vi "C37 Get PMU Configuration.vi"(8 "error in (no error)":errorcluster, 10 "PMU Index":i32, 11 "Pseudo PDC ID":i32) -> (0 "error out":errorcluster, 2 "Station Name":string, 3 "PMU Configuration":T1)   [LabVIEW 2013, in "C37118-DLL.lvlib"]
uses:
  C37118-DLL.lvlib
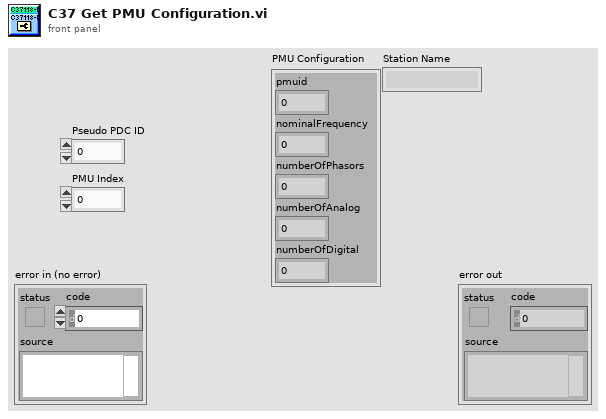
[diagram p1: front panel]
types:
  T1 = cluster{"pmuid":i32, "nominalFrequency":sgl, "numberOfPhasors":i32, "numberOfAnalog":i32, "numberOfDigital":i32}
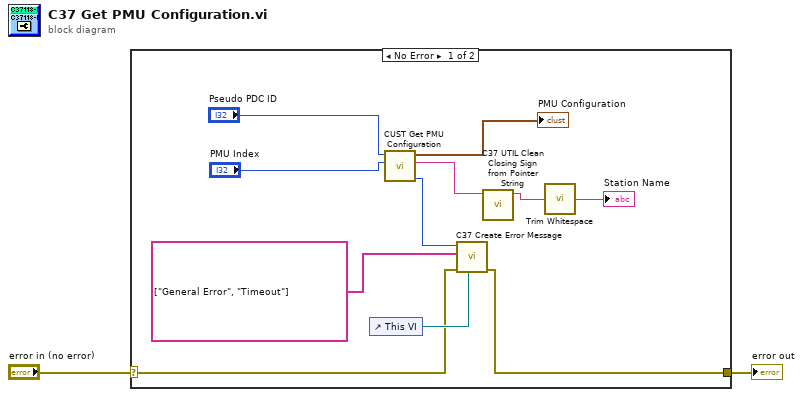
[diagram p0: block diagram]
diagram:
  n1 = case shown="No Error" "error in (no error)" {
    selector: "error in (no error)" -> [w12 w14]
    tunnel: [w11 w14] -> w2
    frame No Error {
      n2 = control-ref of="This VI"() -> (w13:refnum<vi>)
      n3 = call "CUST Get PMU Configuration.vi"("pmuIndex"="PMU Index", "pseudoPdcId"="Pseudo PDC ID") -> ("function return"=w3:i32, "stationName out"=w4:string, "pmuconf out"=→"PMU Configuration":T1)  [unwired: 7 in]
      n4 = call "C37 Create Error Message.vi"("VI Reference"=w13, "error in (no error)"=w12, "Error Messages"=string[] ["General Error", "Timeout"], "function return"=w3) -> ("error out"=w11:errorcluster)  [unwired: 7 in]
      n5 = call "C37 UTIL Clean Closing Sign from Pointer String.vi"("String In"=w4) -> ("String Out"=w8:string)  [unwired: 10 in]
      n6 = call <vilib>:"Trim Whitespace.vi"("string"=w8) -> ("trimmed string"=→"Station Name":string)  [unwired: 1 in]
    }
    frame Error {
    }
  }
  "error out" <- w2
